vi "GetTerm.vi"(8 "error in (no error)":errorcluster, 11 "DefinitionList in":refnum<class "DefinitionList.lvclass">) -> (0 "error out":errorcluster, 2 "Term":string, 3 "DefinitionList out":refnum<class "DefinitionList.lvclass">)   [LabVIEW 2021, in "LvMarkdown.lvlib" / "DefinitionList.lvclass"]
uses:
  DefinitionList.lvclass
  DefinitionList.lvclass/DefinitionList.ctl
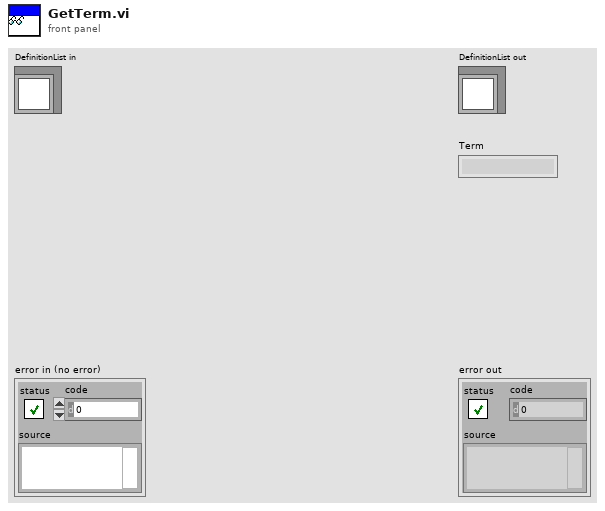
[diagram p1: front panel]
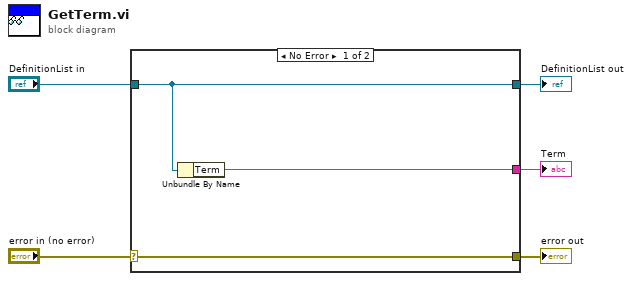
[diagram p0: block diagram]
diagram:
  n1 = case shown="No Error" "error in (no error)" {
    selector: "error in (no error)" -> [w8 w9]
    tunnel: [w8 w9] -> w4
    tunnel: [w7 w10] -> w2
    tunnel: "DefinitionList in" -> [w7 w10]
    tunnel: [w6 _] -> w1
    frame No Error {
      n2 = Unbundle By Name(w7) -> ("Term"=w6:string)
    }
    frame Error {
    }
  }
  "error out" <- w4
  "DefinitionList out" <- w2
  "Term" <- w1
